vi "Get Offline Path.vi"() -> (3 "Offline Path":path=path "NI VeriStand/Custom Device Offline API")   [LabVIEW 2020, in "Custom Device API.lvlib"]
doc: "Reserved for internal use.\n\nThis VI is intended for use only with the Custom Device Offline API."
uses:
  <vilib>/NI VeriStand/Custom Device API/Custom Device API.lvlib
  <vilib>/NI VeriStand/Custom Device API/Custom Device Offline Path.vi
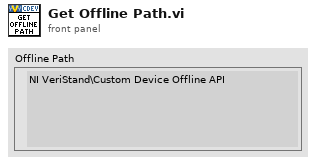
[diagram p1: front panel]
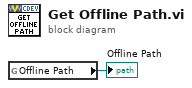
[diagram p0: block diagram]
diagram:
  n1 = global read "Custom Device Offline Path.vi" "Offline Path"() -> (→"Offline Path":path)
